vi "PidHmi.vi"() -> ()   [LabVIEW 2018, in "Pid.lvlib"]
uses:
  Pid.lvlib
  <vilib>/Modbus/master/Create Master Instance (Serial).vi
  <vilib>/Modbus/master/Modbus Master.lvclass
panel:
  in  "Clear Errors":bool
  in  "Tune with time parameters":bool
  in  "Td":sgl
  in  "Ti":sgl
  in  "Kd":sgl
  in  "Ki":sgl
  in  "Kp":sgl
  in  "Force exit out of loop":bool
  in  "Manual":u8(slide) scale=0.0..255.0
  out "Output":i16(knob) scale=0.0..255.0 scale format="%x"
  in  "Stop and close":bool
  in  "Setpoint":sgl(slide) scale=0.0..300.0
  out "Thermometer":sgl(slide) scale=0.0..300.0
  out "Modbus Error":errorcluster
  in  "Serial port":refnum<visa-resource-name>="COM1"
  out "Connected":bool
  in  "Connect to Modbus":bool
  out "Interval":i32
  out "File error":errorcluster
  out "Time":u32
  out "General error":errorcluster
  out "Single Update (Multiple Plots, stacked)":cluster{"Temperature":sgl, "Setpoint":sgl, sgl}(graph)
  out "Cycle":i32
  out "Logging to file":bool
  in  "Start logging to file":bool
  in  "Delimiter":string(combo)
  in  "Format":string(combo)
  in  "Stop the PID":bool
  in  "file path (use dialog)":path
  in  "Frequency":dbl(slide) scale=0.1..10.0
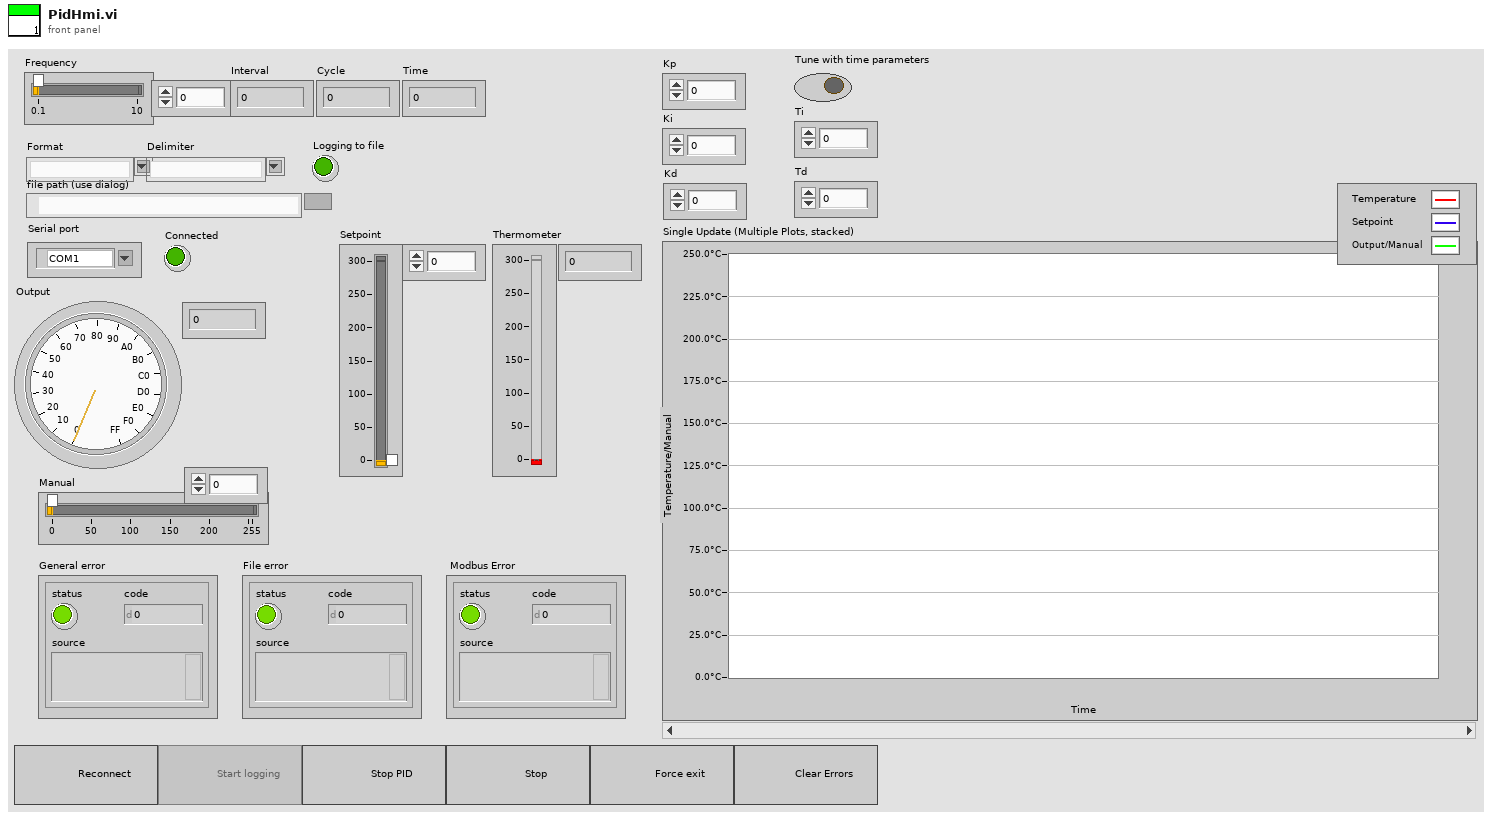
[diagram p1: front panel]
types:
  T1 = enum8{"Enabled", "Disabled", "Disabled and Grayed Out"}
  T2 = enum16{"open", "replace", "create", "open or create", "replace or create", "replace or create with confirmation"}
  T3 = cluster{"Sensor":sgl, "Setpoint":sgl, "Output":sgl}
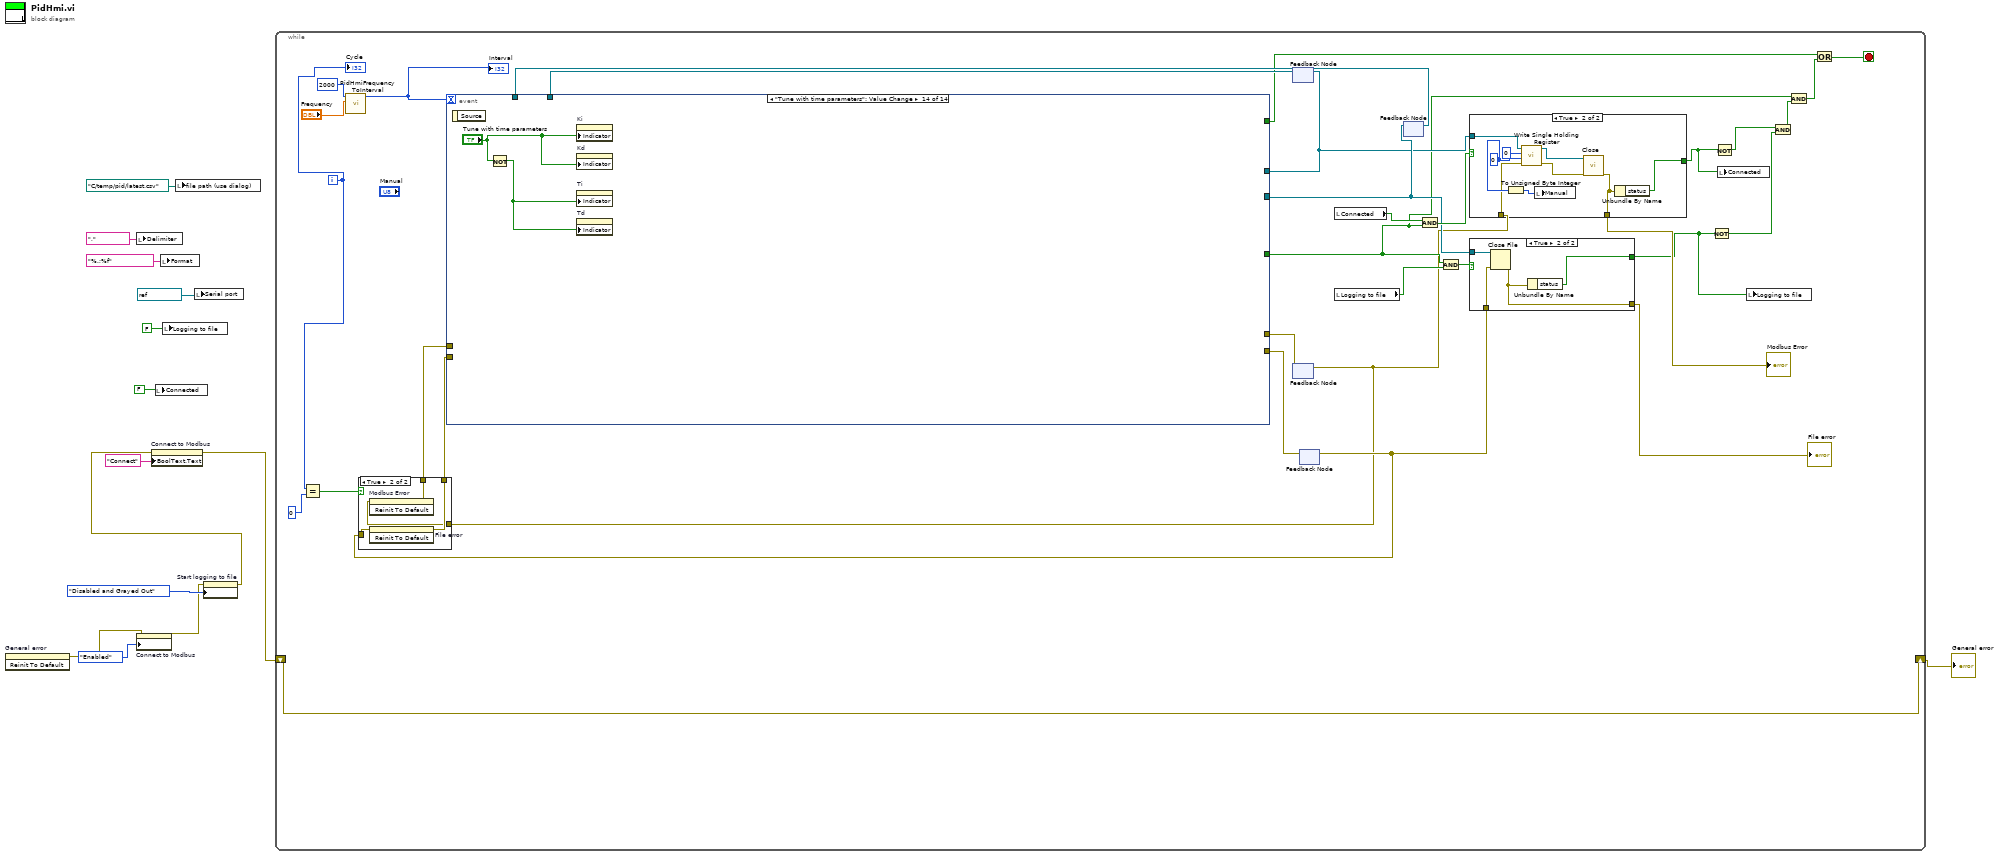
[diagram p0: block diagram]
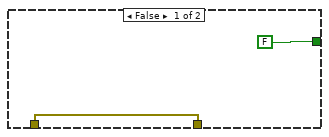
[diagram p3: hidden frame]
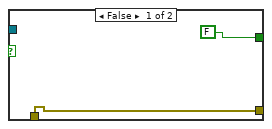
[diagram p4: hidden frame]
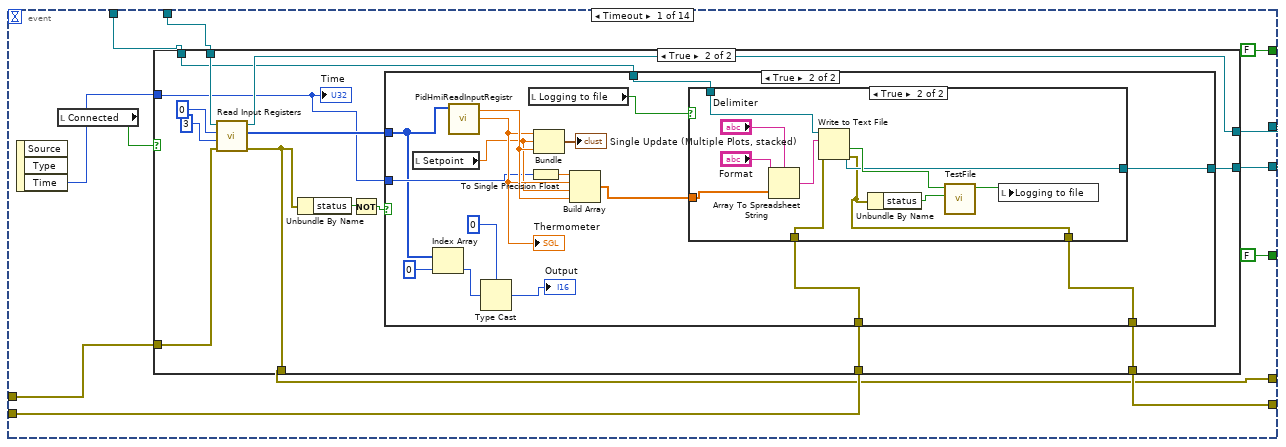
[diagram p5: hidden frame]
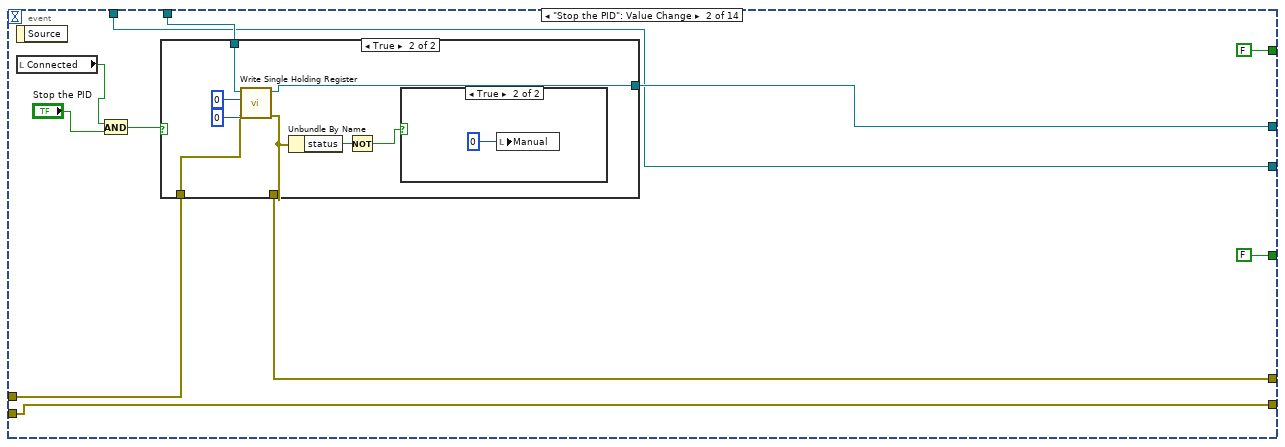
[diagram p9: hidden frame]
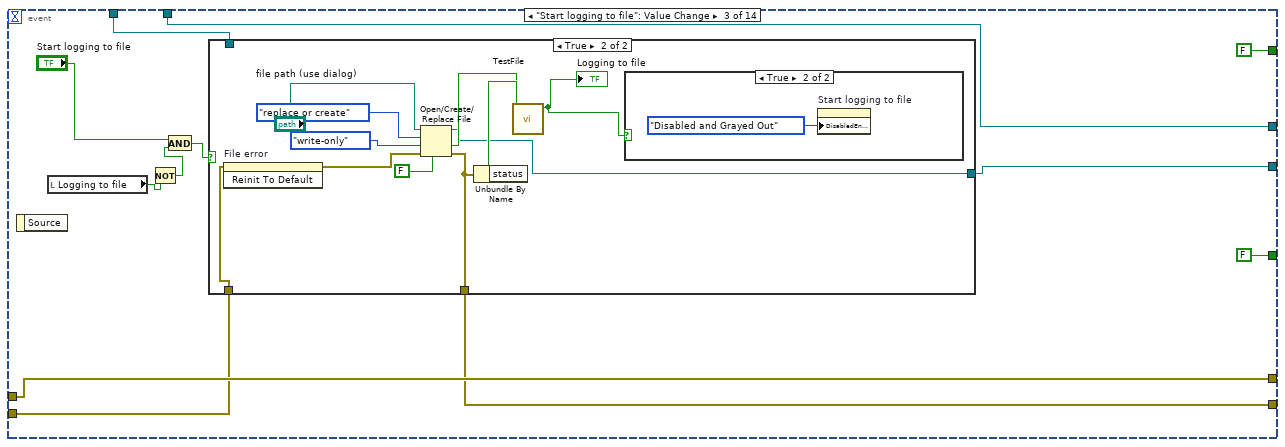
[diagram p12: hidden frame]
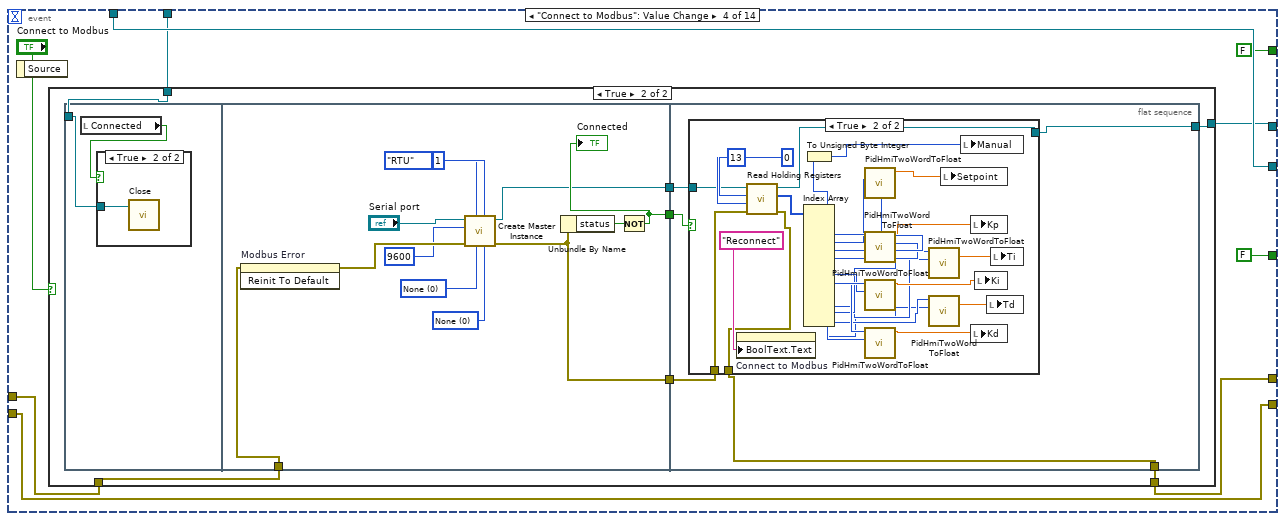
[diagram p15: hidden frame]
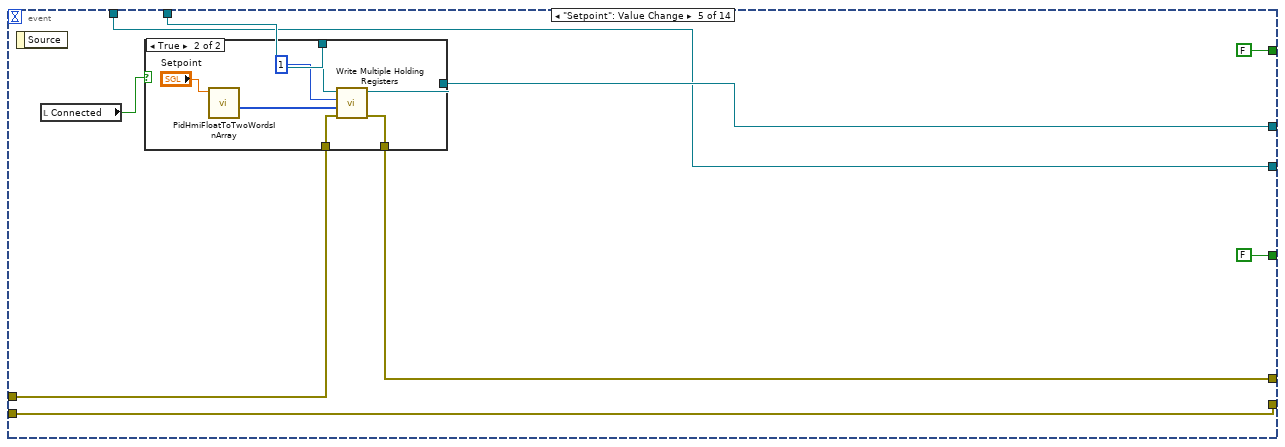
[diagram p19: hidden frame]
diagram:
  n1 = invoke on="General error" class="Clust (strict)" method="Reinit To Default"() -> (error out=w7:errorcluster)  [unwired: 3 in, 2 out]
  n2 = local write "Delimiter"("," ("Delimiter")) -> ()
  n3 = property on="Connect to Modbus" class="Bool"(error in=w7, "DisabledEnum"=T1."Enabled" ("Disabled")) -> (error out=w9:errorcluster)  [unwired: 1 in, 1 out]
  n4 = local write "Connected"(FALSE ("Connected")) -> ()
  n5 = local write "Format"("%.;%f" ("Format")) -> ()
  n6 = local write "Logging to file"(FALSE ("Logging to file")) -> ()
  n7 = local write "file path (use dialog)"(path "C:/temp/pid/latest.csv" ("file path (use dialog)")) -> ()
  n8 = local write "Serial port"(refnum<visa-resource-name> "COM11" ("Serial port")) -> ()
  n9 = property on="Start logging to file" class="Bool"(error in=w9, "DisabledEnum"=T1."Disabled and Grayed Out" ("Disabled")) -> (error out=w1:errorcluster)  [unwired: 1 in, 1 out]
  n10 = property on="Connect to Modbus" class="Bool"(error in=w1, "BoolText.Text"="Connect" ("Boolean Text.Text")) -> (error out=w2:errorcluster)  [unwired: 1 in, 1 out]
  n11 = while {
    shift-right: [w43] -> w5
    shift-left: w2 -> [w43]
    i -> [w22]
    stop <- w27 stop-if-true
    n12 = Equal?(x=w22, y=0) -> (x = y?=w20:bool)
    n13 = call "PidHmiFrequencyToInterval.vi"("Frequence"="Frequency", "Default"=2000) -> ("Numeric"=w44:i32)  [unwired: 9 in]
    "Interval" <- w44
    n14 = feedback #1() -> (w42:refnum<class "Modbus Master.lvclass">)  [unwired: 1 in]
    n15 = feedback #2() -> (w16:errorcluster)  [unwired: 1 in]
    n16 = feedback #3() -> (w18:errorcluster)  [unwired: 1 in]
    n17 = case shown="True" w20 {
      tunnel: [w47 w52] -> w19
      tunnel: w18 -> [w47 w51]
      tunnel: [w48 w50] -> w17
      tunnel: w16 -> [w48 w49]
      frame False {
      }
      frame True {
        n18 = invoke on="Modbus Error" class="Clust (strict)" method="Reinit To Default"(error in=w49) -> (error out=w50:errorcluster)  [unwired: 2 in, 2 out]
        n19 = invoke on="File error" class="Clust (strict)" method="Reinit To Default"(error in=w51) -> (error out=w52:errorcluster)  [unwired: 2 in, 2 out]
      }
    }
    n20 = local read "Connected"() -> (w36:bool)
    n21 = local read "Logging to file"() -> (w38:bool)
    n22 = feedback #4() -> (w41:refnum<file>)  [unwired: 1 in]
    n23 = event shown="[13] \"Tune with time parameters\": Value Change" {
      selector: _ -> [_ _ _ _ _ _ _ _ _ _ _ _ _ _]
      dyn-events: _ -> [_ _ _ _ _ _ _ _ _ _ _ _ _ _]
      timeout: w44 -> [_ _ _ _ _ _ _ _ _ _ _ _ _ _]
      tunnel: [w80 w134 w157 w187 w250 w269 w276 w283 w298 w313 w330 w347 w365 _] -> w33
      tunnel: [w73 w142 w158 w188 w251 w271 w274 w286 w302 w315 w334 w351 w370 _] -> w40
      tunnel: [w79 w137 w165 w180 w253 w268 w277 w278 w299 w314 w331 w350 w368 _] -> w32
      tunnel: w42 -> [w77 w138 w165 w183 w255 w268 w277 w281 w299 w317 w336 w354 w372 _]
      tunnel: w41 -> [w76 w134 w156 w187 w250 w269 w276 w283 w298 w313 w330 w347 w365 _]
      tunnel: [w72 w135 w164 w181 w254 w270 w275 w279 w300 w316 w335 w352 w369 _] -> w39
      tunnel: w19 -> [w74 w142 w159 w188 w251 w271 w274 w286 w303 w315 w334 w351 w370 _]
      tunnel: w17 -> [w75 w136 w164 w182 w252 w270 w275 w280 w301 w318 w337 w353 w371 _]
      tunnel: [FALSE ("Stop and close") FALSE ("Stop and close") FALSE ("Stop and close") FALSE ("Stop and close") FALSE ("Stop and close") "Stop and close" FALSE ("Stop and close") FALSE ("Stop and close") FALSE ("Stop and close") FALSE ("Stop and close") FALSE ("Stop and close") FALSE ("Stop and close") FALSE ("Stop and close") _] -> w24
      tunnel: [FALSE ("Force exit out of loop") FALSE ("Force exit out of loop") FALSE ("Force exit out of loop") FALSE ("Force exit out of loop") FALSE ("Force exit out of loop") FALSE ("Force exit out of loop") "Force exit out of loop" FALSE ("Force exit out of loop") FALSE ("Force exit out of loop") FALSE ("Force exit out of loop") FALSE ("Force exit out of loop") FALSE ("Force exit out of loop") FALSE ("Force exit out of loop") _] -> w23
      event Timeout {
        n24 = event-data() -> ("Time"=w78:u32)  [unwired: 1 in, 2 out]
        n25 = local read "Connected"() -> (w81:bool)
        n26 = case shown="True" w81 {
          tunnel: [w84 w96] -> w80
          tunnel: w78 -> [_ w88]
          tunnel: [w85 w90] -> w79
          tunnel: w77 -> [w85 w95]
          tunnel: w76 -> [w84 w89]
          tunnel: w75 -> [w83 w94]
          tunnel: w74 -> [w82 w93]
          tunnel: [w82 w92] -> w73
          tunnel: [w83 w91] -> w72
          frame False {
          }
          frame True {
            n27 = call-dynamic "Read Input Registers.vi"("error in (no error)"=w94, "number of input registers"=u16 3, "starting address"=u16 0, "Modbus master in"=w95) -> ("error out"=w91:errorcluster, "register values"=w97:u16[], "Modbus master out"=w90:refnum<class "Modbus Master.lvclass">)  [unwired: 5 in]
            n28 = Unbundle By Name(w91) -> ("status"=w87:bool)
            n29 = Not(x=w87) -> (.not. x?=w86:bool)
            n30 = case shown="True" w86 {
              tunnel: w97 -> [_ w106]
              tunnel: [w100 w117] -> w96
              tunnel: w93 -> [w101 w113]
              tunnel: [w101 w112] -> w92
              tunnel: w89 -> [w100 w109]
              tunnel: w88 -> [_ w107]
              frame False {
              }
              frame True {
                n31 = local read "Setpoint"() -> (w108:sgl)
                n32 = Index Array(array=w106, index=0) -> (element=w103:u16)
                n33 = call "PidHmiReadInputRegistr.vi"("register values"=w106) -> ("Sensor"=w114:sgl, "Output"=w118:sgl)  [unwired: 9 in]
                "Thermometer" <- w114
                n34 = Type Cast(type=i16 0 ("Output"), x=w103) -> (*(type *) &x=→"Output":i16)
                n35 = local read "Logging to file"() -> (w111:bool)
                n36 = To Single Precision Float(number=w107) -> (single precision float=w115:sgl)
                n37 = Bundle("Sensor"=w114, "Setpoint"=w108, "Output"=w118) -> (→"Single Update (Multiple Plots, stacked)":T3)  [unwired: 1 in]
                n38 = Build Array(w115, w114, w108, w118) -> (w110:sgl[])
                n39 = case shown="True" w111 {
                  tunnel: [w119 w126] -> w117
                  tunnel: w110 -> [_ w124]
                  tunnel: [w120 w123] -> w112
                  tunnel: w113 -> [w120 w122]
                  tunnel: w109 -> [w119 w121]
                  frame False {
                  }
                  frame True {
                    n40 = Array To Spreadsheet String(delimiter (Tab)="Delimiter", array=w124, 3:"Format") -> (spreadsheet string=w131:string)
                    n41 = Write to Text File(file (use dialog)=w121, text=w131, error in=w122) -> (refnum out=w126:refnum<file>, cancelled=w130:bool, error out=w123:errorcluster)  [unwired: 1 in]
                    n42 = Unbundle By Name(w123) -> ("status"=w129:bool)
                    n43 = call "TestFile.vi"("status"=w129, "cancelled"=w130) -> ("IsOpen"=w125:bool)  [unwired: 9 in]
                    n44 = local write "Logging to file"(w125) -> ()
                  }
                }
              }
            }
            "Time" <- w88
          }
        }
      }
      event "Stop the PID": Value Change {
        n45 = event-data() -> ()  [unwired: 1 in, 1 out]
        n46 = local read "Connected"() -> (w141:bool)
        n47 = And(x=w141, y="Stop the PID") -> (x .and. y?=w139:bool)
        n48 = case shown="True" w139 {
          tunnel: w138 -> [w143 w152]
          tunnel: [w143 w151] -> w137
          tunnel: w136 -> [w144 w148]
          tunnel: [w144 w147] -> w135
          frame False {
          }
          frame True {
            n49 = call-dynamic "Write Single Holding Register.vi"("error in (no error)"=w148, "holding register value"=u16 0, "address"=u16 0, "Modbus master in"=w152) -> ("error out"=w147:errorcluster, "Modbus master out"=w151:refnum<class "Modbus Master.lvclass">)  [unwired: 6 in]
            n50 = Unbundle By Name(w147) -> ("status"=w146:bool)
            n51 = Not(x=w146) -> (.not. x?=w145:bool)
            n52 = case shown="True" w145 {
              frame False {
              }
              frame True {
                n53 = local write "Manual"(u8 0 ("Manual")) -> ()
              }
            }
          }
        }
      }
      event "Start logging to file": Value Change {
        n54 = event-data() -> ()  [unwired: 1 in, 1 out]
        n55 = local read "Logging to file"() -> (w163:bool)
        n56 = Not(x=w163) -> (.not. x?=w162:bool)
        n57 = And(x="Start logging to file", y=w162) -> (x .and. y?=w160:bool)
        n58 = case shown="True" w160 {
          tunnel: w159 -> [w167 w171]
          tunnel: [w167 w170] -> w158
          tunnel: [w166 w168] -> w157
          tunnel: w156 -> [w166 _]
          frame False {
          }
          frame True {
            n59 = invoke on="File error" class="Clust (strict)" method="Reinit To Default"(error in=w171) -> (error out=w175:errorcluster)  [unwired: 2 in, 2 out]
            n60 = Open/Create/Replace File(file path (use dialog)="file path (use dialog)", error in=w175, operation (0:open)=T2."replace or create", access (0:read/write)=enum16{"read/write", "read-only", "write-only"}."write-only", disable buffering (F)=FALSE) -> (refnum out=w168:refnum<file>, cancelled=w177:bool, error out=w170:errorcluster)  [unwired: 1 in]
            n61 = Unbundle By Name(w170) -> ("status"=w178:bool)
            n62 = call "TestFile.vi"("status"=w178, "cancelled"=w177) -> ("IsOpen"=w169:bool)  [unwired: 9 in]
            "Logging to file" <- w169
            n63 = case shown="True" w169 {
              frame False {
              }
              frame True {
                n64 = property on="Start logging to file" class="Bool"("DisabledEnum"=T1."Disabled and Grayed Out" ("Disabled")) -> ()  [unwired: 2 in, 2 out]
              }
            }
          }
        }
      }
      event "Connect to Modbus": Value Change {
        n65 = event-data() -> ()  [unwired: 1 in, 1 out]
        n66 = case shown="True" "Connect to Modbus" {
          tunnel: w183 -> [w190 w197]
          tunnel: w182 -> [w189 w196]
          tunnel: [w189 w192] -> w181
          tunnel: [w190 w191] -> w180
          frame False {
          }
          frame True {
            n67 = flat-sequence {
              tunnel: w197 -> [w199]
              tunnel: w196 -> [w204]
              tunnel: [w203] -> w195
              tunnel: [w202] -> w194
              tunnel: [w201] -> w193
              tunnel: w195 -> [w217]
              tunnel: w194 -> [w216]
              tunnel: w193 -> [w215]
              tunnel: [w214] -> w192
              tunnel: [w213] -> w191
              frame #0 {
                n68 = local read "Connected"() -> (w198:bool)
                n69 = case shown="True" w198 {
                  tunnel: w199 -> [_ w200]
                  frame False {
                  }
                  frame True {
                    n70 = call-dynamic "Close.vi"("Modbus master in"=w200) -> ()  [unwired: 10 in, 1 out]
                  }
                }
              }
              frame #1 {
                w209 = u16 0 items=["None", "XON/XOFF", "RTS/CTS", "XON/XOFF & RTS/CTS", "DTR/DSR", "XON/XOFF & DTR/DSR"] ("flow control (None)")
                w207 = u16 0 items=["None", "Odd", "Even"] ("parity (Even)")
                n71 = invoke on="Modbus Error" class="Clust (strict)" method="Reinit To Default"(error in=w204) -> (error out=w210:errorcluster)  [unwired: 2 in, 2 out]
                n72 = call-poly <vilib>:"Create Master Instance.vi"("flow control (None)"=w209, "serial type"=enum16{"RTU", "ASCII"}."RTU", "parity (Even)"=w207, "unit ID"=u8 1, "error in (no error)"=w210, "baud rate (9600)"=u32 9600, "VISA resource name"="Serial port") -> ("error out"=w202:errorcluster, "serial master instance"=w201:refnum<class "Modbus Master.lvclass">)  [unwired: 3 in]
                n73 = Unbundle By Name(w202) -> ("status"=w212:bool)
                n74 = Not(x=w212) -> (.not. x?=w203:bool)
                "Connected" <- w203
              }
              frame #2 {
                n75 = case shown="True" w217 {
                  tunnel: w216 -> [w218 w223]
                  tunnel: w215 -> [w219 w222]
                  tunnel: [w218 w221] -> w214
                  tunnel: [w219 w220] -> w213
                  frame False {
                  }
                  frame True {
                    n76 = property on="Connect to Modbus" class="Bool"("BoolText.Text"="Reconnect" ("Boolean Text.Text")) -> ()  [unwired: 2 in, 2 out]
                    n77 = call-dynamic "Read Holding Registers.vi"("error in (no error)"=w223, "number of holding registers"=u16 13, "starting address"=u16 0, "Modbus master in"=w222) -> ("error out"=w221:errorcluster, "register values"=w245:u16[], "Modbus master out"=w220:refnum<class "Modbus Master.lvclass">)  [unwired: 5 in]
                    n78 = Index Array(array=w245) -> (element #1=w240:u16, element #2=w243:u16, element #3=w242:u16, element #4=w239:u16, element #5=w238:u16, element #6=w236:u16, element #7=w235:u16, element #8=w233:u16, element #9=w232:u16, element #10=w230:u16, element #11=w229:u16, element #12=w227:u16, element #13=w226:u16)  [unwired: 13 in]
                    n79 = To Unsigned Byte Integer(number=w240) -> (unsigned 8bit integer=w241:u8)
                    n80 = call "PidHmiTwoWordToFloat.vi"("register 2"=w242, "register 1"=w243) -> ("number"=w244:sgl)  [unwired: 9 in]
                    n81 = call "PidHmiTwoWordToFloat.vi"("register 2"=w238, "register 1"=w239) -> ("number"=w237:sgl)  [unwired: 9 in]
                    n82 = call "PidHmiTwoWordToFloat.vi"("register 2"=w235, "register 1"=w236) -> ("number"=w234:sgl)  [unwired: 9 in]
                    n83 = call "PidHmiTwoWordToFloat.vi"("register 2"=w232, "register 1"=w233) -> ("number"=w231:sgl)  [unwired: 9 in]
                    n84 = call "PidHmiTwoWordToFloat.vi"("register 2"=w229, "register 1"=w230) -> ("number"=w228:sgl)  [unwired: 9 in]
                    n85 = call "PidHmiTwoWordToFloat.vi"("register 2"=w226, "register 1"=w227) -> ("number"=w225:sgl)  [unwired: 9 in]
                    n86 = local write "Setpoint"(w244) -> ()
                    n87 = local write "Manual"(w241) -> ()
                    n88 = local write "Kp"(w237) -> ()
                    n89 = local write "Kd"(w231) -> ()
                    n90 = local write "Ki"(w234) -> ()
                    n91 = local write "Td"(w225) -> ()
                    n92 = local write "Ti"(w228) -> ()
                  }
                }
              }
            }
          }
        }
      }
      event "Setpoint": Value Change {
        n93 = event-data() -> ()  [unwired: 1 in, 1 out]
        n94 = local read "Connected"() -> (w256:bool)
        n95 = case shown="True" w256 {
          tunnel: w255 -> [w258 w264]
          tunnel: [w258 w261] -> w253
          tunnel: [w257 w260] -> w254
          tunnel: w252 -> [w257 w259]
          frame False {
          }
          frame True {
            n96 = call "PidHmiFloatToTwoWordsInArray.vi"("Float"="Setpoint") -> ("TwoWordArray"=w262:u16[])  [unwired: 10 in]
            n97 = call-dynamic "Write Multiple Holding Registers.vi"("error in (no error)"=w259, "holding register values"=w262, "starting address"=u16 1, "Modbus master in"=w264) -> ("error out"=w260:errorcluster, "Modbus master out"=w261:refnum<class "Modbus Master.lvclass">)  [unwired: 6 in]
          }
        }
      }
      event "Stop and close": Value Change {
        n98 = event-data() -> ()  [unwired: 1 in, 1 out]
      }
      event "Force exit out of loop": Value Change {
        n99 = event-data() -> ()  [unwired: 1 in, 1 out]
      }
      event "Kp": Value Change {
        n100 = event-data() -> ()  [unwired: 1 in, 1 out]
        n101 = local read "Connected"() -> (w282:bool)
        n102 = case shown="True" w282 {
          tunnel: [w288 w293] -> w278
          tunnel: [w287 w292] -> w279
          tunnel: w281 -> [w288 w290]
          tunnel: w280 -> [w287 w289]
          frame False {
          }
          frame True {
            n103 = call "PidHmiFloatToTwoWordsInArray.vi"("Float"="Kp") -> ("TwoWordArray"=w294:u16[])  [unwired: 10 in]
            n104 = call-dynamic "Write Multiple Holding Registers.vi"("error in (no error)"=w289, "holding register values"=w294, "starting address"=u16 3, "Modbus master in"=w290) -> ("error out"=w292:errorcluster, "Modbus master out"=w293:refnum<class "Modbus Master.lvclass">)  [unwired: 6 in]
          }
        }
      }
      event "Clear Errors": Value Change {
        n105 = event-data() -> ()  [unwired: 1 in, 1 out]
        n106 = case shown="True" "Clear Errors" {
          tunnel: w303 -> [w306 w310]
          tunnel: [w306 w309] -> w302
          tunnel: w301 -> [w305 w308]
          tunnel: [w305 w307] -> w300
          frame False {
          }
          frame True {
            n107 = invoke on="Modbus Error" class="Clust (strict)" method="Reinit To Default"(error in=w308) -> (error out=w307:errorcluster)  [unwired: 2 in, 2 out]
            n108 = invoke on="File error" class="Clust (strict)" method="Reinit To Default"(error in=w310) -> (error out=w309:errorcluster)  [unwired: 2 in, 2 out]
          }
        }
      }
      event "Ki": Value Change {
        n109 = event-data() -> ()  [unwired: 1 in, 1 out]
        n110 = local read "Connected"() -> (w319:bool)
        n111 = case shown="False" w319 {
          tunnel: [w320 w326] -> w314
          tunnel: [w321 w325] -> w316
          tunnel: w318 -> [w321 w323]
          tunnel: w317 -> [w320 w322]
          frame False {
          }
          frame True {
            n112 = call "PidHmiFloatToTwoWordsInArray.vi"("Float"="Ki") -> ("TwoWordArray"=w327:u16[])  [unwired: 10 in]
            n113 = call-dynamic "Write Multiple Holding Registers.vi"("error in (no error)"=w323, "holding register values"=w327, "starting address"=u16 5, "Modbus master in"=w322) -> ("error out"=w325:errorcluster, "Modbus master out"=w326:refnum<class "Modbus Master.lvclass">)  [unwired: 6 in]
          }
        }
      }
      event "Kd": Value Change {
        n114 = local read "Connected"() -> (w329:bool)
        n115 = event-data() -> ()  [unwired: 1 in, 1 out]
        n116 = case shown="False" w329 {
          tunnel: [w338 w344] -> w331
          tunnel: [w339 w343] -> w335
          tunnel: w337 -> [w339 w341]
          tunnel: w336 -> [w338 w340]
          frame False {
          }
          frame True {
            n117 = call "PidHmiFloatToTwoWordsInArray.vi"("Float"="Kd") -> ("TwoWordArray"=w345:u16[])  [unwired: 10 in]
            n118 = call-dynamic "Write Multiple Holding Registers.vi"("error in (no error)"=w341, "holding register values"=w345, "starting address"=u16 7, "Modbus master in"=w340) -> ("error out"=w343:errorcluster, "Modbus master out"=w344:refnum<class "Modbus Master.lvclass">)  [unwired: 6 in]
          }
        }
      }
      event "Ti": Value Change {
        n119 = event-data() -> ()  [unwired: 1 in, 1 out]
        n120 = local read "Connected"() -> (w355:bool)
        n121 = case shown="False" w355 {
          tunnel: [w356 w362] -> w350
          tunnel: [w357 w361] -> w352
          tunnel: w354 -> [w356 w359]
          tunnel: w353 -> [w357 w358]
          frame False {
          }
          frame True {
            n122 = call "PidHmiFloatToTwoWordsInArray.vi"("Float"="Ti") -> ("TwoWordArray"=w363:u16[])  [unwired: 10 in]
            n123 = call-dynamic "Write Multiple Holding Registers.vi"("error in (no error)"=w358, "holding register values"=w363, "starting address"=u16 9, "Modbus master in"=w359) -> ("error out"=w361:errorcluster, "Modbus master out"=w362:refnum<class "Modbus Master.lvclass">)  [unwired: 6 in]
          }
        }
      }
      event "Td": Value Change {
        n124 = event-data() -> ()  [unwired: 1 in, 1 out]
        n125 = local read "Connected"() -> (w373:bool)
        n126 = case shown="False" w373 {
          tunnel: [w375 w380] -> w368
          tunnel: [w374 w379] -> w369
          tunnel: w372 -> [w375 w377]
          tunnel: w371 -> [w374 w376]
          frame False {
          }
          frame True {
            n127 = call "PidHmiFloatToTwoWordsInArray.vi"("Float"="Td") -> ("TwoWordArray"=w381:u16[])  [unwired: 10 in]
            n128 = call-dynamic "Write Multiple Holding Registers.vi"("error in (no error)"=w376, "holding register values"=w381, "starting address"=u16 11, "Modbus master in"=w377) -> ("error out"=w379:errorcluster, "Modbus master out"=w380:refnum<class "Modbus Master.lvclass">)  [unwired: 6 in]
          }
        }
      }
      event "Tune with time parameters": Value Change {
        n129 = event-data() -> ()  [unwired: 1 in, 1 out]
        n130 = Not(x="Tune with time parameters") -> (.not. x?=w383:bool)
        n131 = property on="Ki" class="DigNum (strict)"("Indicator"="Tune with time parameters") -> ()  [unwired: 2 in, 2 out]
        n132 = property on="Kd" class="DigNum (strict)"("Indicator"="Tune with time parameters") -> ()  [unwired: 2 in, 2 out]
        n133 = property on="Ti" class="DigNum (strict)"("Indicator"=w383) -> ()  [unwired: 2 in, 2 out]
        n134 = property on="Td" class="DigNum (strict)"("Indicator"=w383) -> ()  [unwired: 2 in, 2 out]
      }
    }
    n135 = feedback-in #1(w32) -> ()
    n136 = feedback-in #2(w39) -> ()
    n137 = feedback-in #3(w40) -> ()
    n138 = feedback-in #4(w33) -> ()
    n139 = And(x=w36, y=w24) -> (x .and. y?=w35:bool)
    n140 = And(x=w24, y=w38) -> (x .and. y?=w37:bool)
    n141 = case shown="True" w35 {
      tunnel: [FALSE w55] -> w15
      tunnel: [w53 w60] -> w31
      tunnel: w32 -> [_ w57]
      tunnel: w16 -> [w53 w56]
      frame False {
      }
      frame True {
        w58 = u16 0 ("holding register value")
        n142 = To Unsigned Byte Integer(number=w58) -> (unsigned 8bit integer=w59:u8)
        n143 = call-dynamic "Write Single Holding Register.vi"("error in (no error)"=w56, "holding register value"=w58, "address"=u16 0, "Modbus master in"=w57) -> ("error out"=w63:errorcluster, "Modbus master out"=w62:refnum<class "Modbus Master.lvclass">)  [unwired: 6 in]
        n144 = local write "Manual"(w59) -> ()
        n145 = call-dynamic "Close.vi"("error in (no error)"=w63, "Modbus master in"=w62) -> ("error out"=w60:errorcluster)  [unwired: 9 in]
        n146 = Unbundle By Name(w60) -> ("status"=w55:bool)
      }
    }
    "Modbus Error" <- w31
    n147 = case shown="True" w37 {
      tunnel: [w65 w69] -> w34
      tunnel: w18 -> [w65 w68]
      tunnel: w33 -> [_ w67]
      tunnel: [FALSE w66] -> w30
      frame False {
      }
      frame True {
        n148 = Close File(refnum=w67, error in=w68) -> (error out=w69:errorcluster)  [unwired: 1 out]
        n149 = Unbundle By Name(w69) -> ("status"=w66:bool)
      }
    }
    "File error" <- w34
    n150 = Not(x=w30) -> (.not. x?=w28:bool)
    n151 = Not(x=w15) -> (.not. x?=w29:bool)
    n152 = local write "Connected"(w15) -> ()
    n153 = local write "Logging to file"(w30) -> ()
    n154 = And(x=w29, y=w28) -> (x .and. y?=w26:bool)
    n155 = And(x=w24, y=w26) -> (x .and. y?=w25:bool)
    n156 = Or(x=w23, y=w25) -> (x .or. y?=w27:bool)
    "Cycle" <- w22
  }
  "General error" <- w5
